vi "Get Frames.vi"(8 "error in (no error)":errorcluster, 10 "Action":T2, 11 "Custom Device reference in":refnum<k24>) -> (0 "error out":errorcluster, 2 "Frame Array":T1[](array[typedef]), 3 "Custom Device reference out":refnum<k24>)   [LabVIEW 2013, in "J1939 System Definition API Support.lvlib"]
uses:
  J1939 System Definition API Support.lvlib
  NationalInstruments.VeriStand.SystemDefinitionAPI
  Types/Remove Frame Action.ctl
  Types/Remove Item - Frame Cluster.ctl
  Shared/SubVIs/Constants.vi
  <vilib>/NI Veristand/Custom Device Tools/Custom Device Utility Library/NI VeriStand - Search for Item by GUID.vi
  <vilib>/NI Veristand/Custom Device Tools/Custom Device Utility Library/Custom Device Utility Library.lvlib
  Shared/J1939 Addon Shared.lvlib
  <vilib>/NI Veristand/Custom Device API/Custom Device API.lvlib
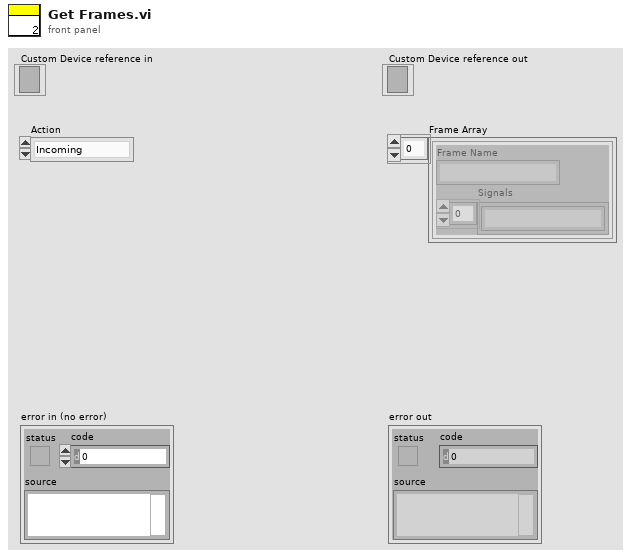
[diagram p1: front panel]
types:
  T1 = typedef "J1939 System Definition API Support.lvlib/Remove Item - Frame Cluster.ctl" = cluster{"Frame Name":string, "Signals":string[]}
  T2 = typedef "J1939 System Definition API Support.lvlib/Remove Frame Action.ctl" = enum16{"Incoming", "Outgoing"}
  T3 = typedef "Custom Device API.lvlib/Custom Device Item Ref.ctl" = u64
  T4 = typedef "Custom Device API.lvlib/Custom Device Item Info.ctl" = cluster{"Name":string, "Is Channel":bool, "GUID":string, "Is Waveform":bool}
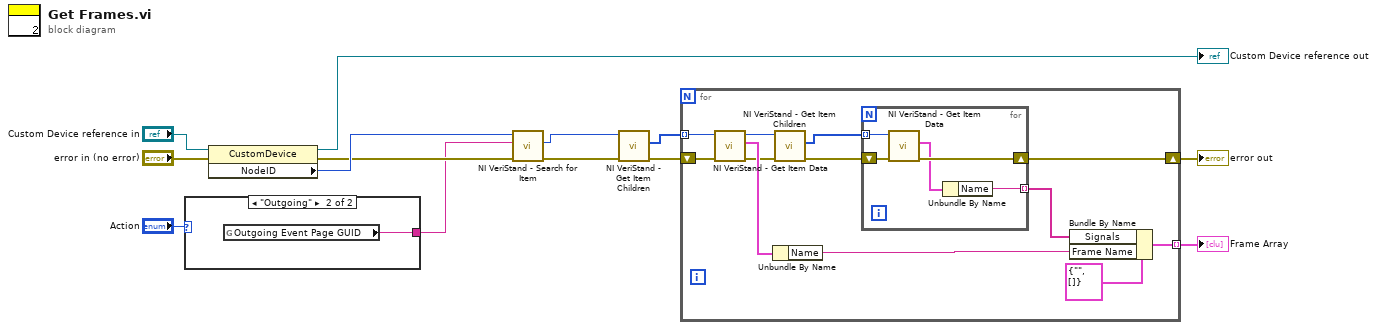
[diagram p0: block diagram]
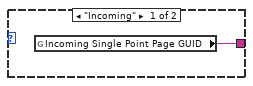
[diagram p2: hidden frame]
diagram:
  n1 = case shown="\"Outgoing\"" "Action" {
    tunnel: [w14 w15] -> w7
    frame "Incoming" {
      n2 = global read "Constants.vi" "Incoming Single Point Page GUID"() -> (w14:string)
    }
    frame "Outgoing" {
      n3 = global read "Constants.vi" "Outgoing Event Page GUID"() -> (w15:string)
    }
  }
  n4 = property class="CustomDevice"(reference="Custom Device reference in", error in="error in (no error)") -> (reference out=→"Custom Device reference out":refnum<k24>, error out=w12:errorcluster, "NodeID"=w13:u64)
  n5 = call-poly <vilib>:"NI VeriStand - Search for Item.vi"("error in"=w12, "Item GUID"=w7, "Section Ref in"=w13) -> ("error out"=w5:errorcluster, "Item Ref"=w6:T3)  [unwired: 5 in, 2 out]
  n6 = call <vilib>:"NI VeriStand - Get Item Children.vi"("error in (no error)"=w5, "Item Ref in"=w6) -> ("error out"=w4:errorcluster, "Child Refs"=w3:T3[])  [unwired: 6 in, 2 out]
  n7 = for {
    tunnel: w3 -> [w25] mode=indexing
    shift-right: [w20] -> w2
    shift-left: w4 -> [w27]
    tunnel: [w16] -> w1 mode=indexing
    n8 = call <vilib>:"NI VeriStand - Get Item Data.vi"("error in (no error)"=w27, "Item Ref in"=w25) -> ("error out"=w24:errorcluster, "Item Info"=w26:T4, "Item Ref out"=w23:T3)  [unwired: 6 in, 1 out]
    n9 = Unbundle By Name(w26) -> ("Name"=w18:string)
    n10 = call <vilib>:"NI VeriStand - Get Item Children.vi"("error in (no error)"=w24, "Item Ref in"=w23) -> ("error out"=w21:errorcluster, "Child Refs"=w22:T3[])  [unwired: 6 in, 2 out]
    n11 = for {
      tunnel: w22 -> [w32] mode=indexing
      shift-right: [w30] -> w20
      shift-left: w21 -> [w31]
      tunnel: [w28] -> w17 mode=indexing
      n12 = call <vilib>:"NI VeriStand - Get Item Data.vi"("error in (no error)"=w31, "Item Ref in"=w32) -> ("error out"=w30:errorcluster, "Item Info"=w29:T4)  [unwired: 6 in, 2 out]
      n13 = Unbundle By Name(w29) -> ("Name"=w28:string)
    }
    n14 = Bundle By Name(cluster=T1 {"Frame Name"="", "Signals"=[]} ("Cluster"), "Signals"=w17, "Frame Name"=w18) -> (w16:T1)
  }
  "error out" <- w2
  "Frame Array" <- w1
